vi "CFG Convert String to DAQ Terminal.vi"(5 "VISA String":string) -> (2 "Terminal":tag)   [LabVIEW 2012]
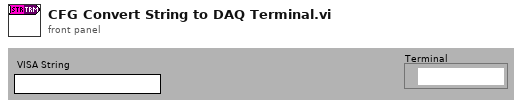
[diagram p1: front panel]
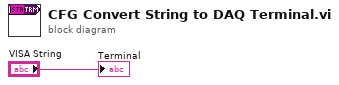
[diagram p0: block diagram]
diagram:
  "Terminal" <- "VISA String"
